vi "Move_Copy.vi"(1 "Mode":enum16{"Move", "Copy"}(ring), 2 "Send error message?":bool=TRUE, 3 "Only Local Copy?":bool, 4 "target path":path, 6 "source path":path) -> ()   [LabVIEW 2010]
uses:
  Update_Global.vi
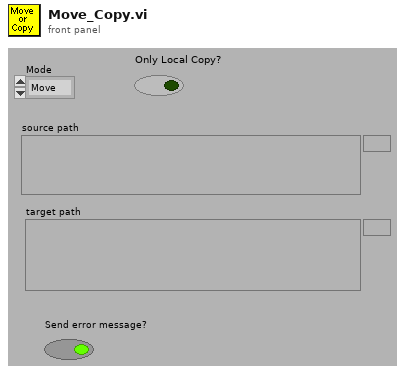
[diagram p1: front panel]
types:
  T1 = enum16{"read/write", "read-only", "write-only", "write-only (truncate)"}
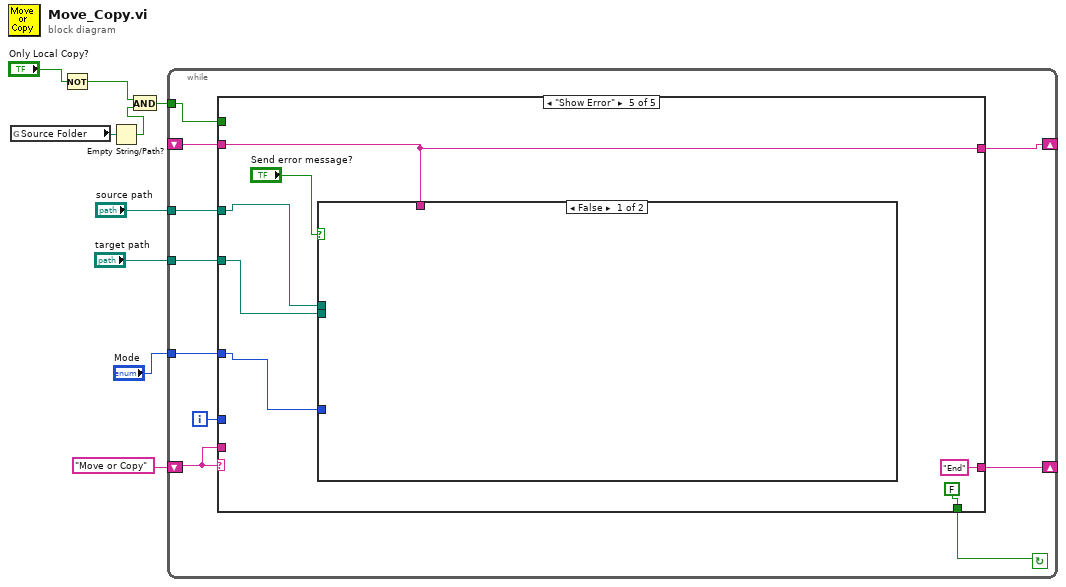
[diagram p0: block diagram]
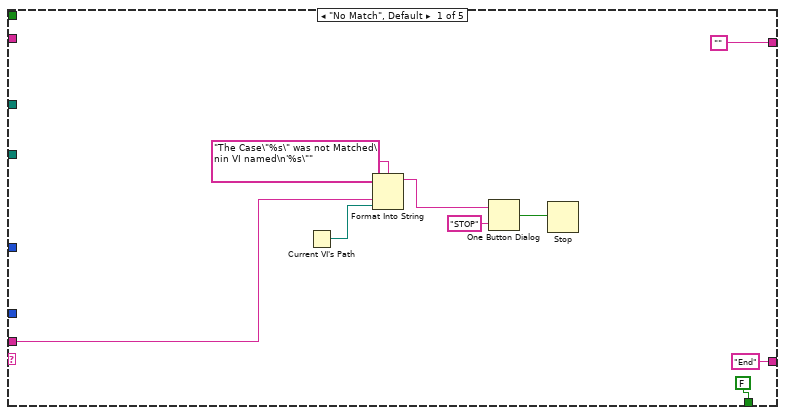
[diagram p2: hidden frame]
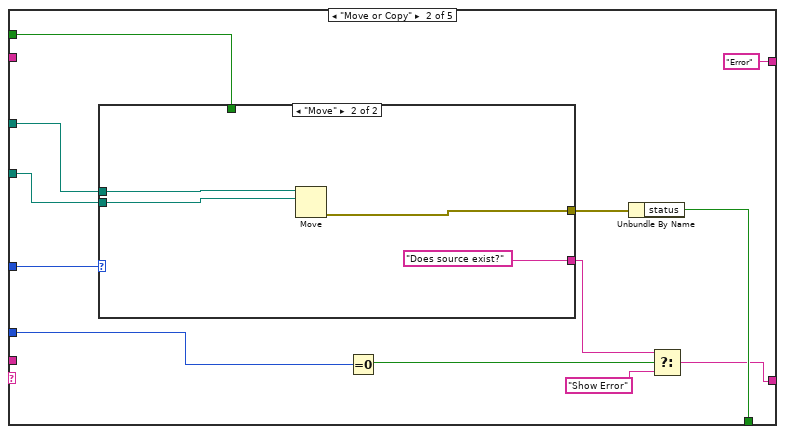
[diagram p3: hidden frame]
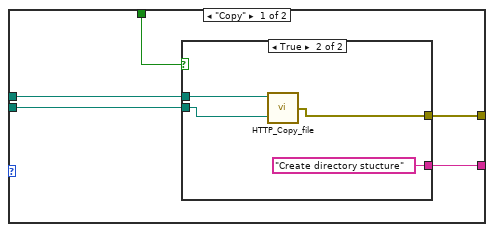
[diagram p4: hidden frame]
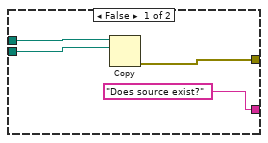
[diagram p5: hidden frame]
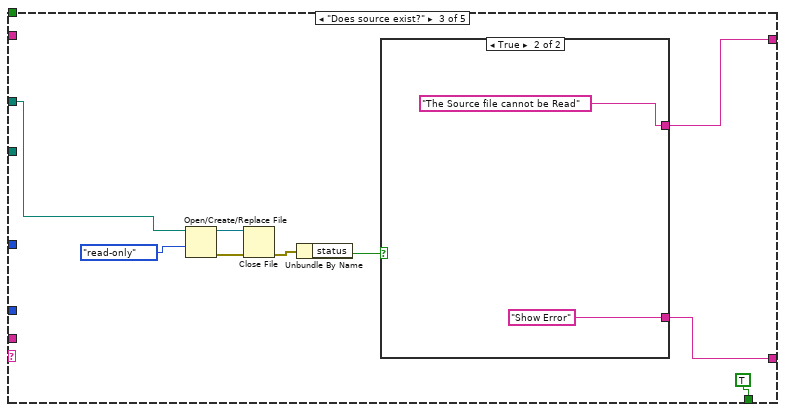
[diagram p6: hidden frame]
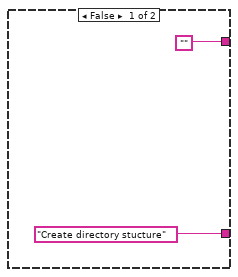
[diagram p7: hidden frame]
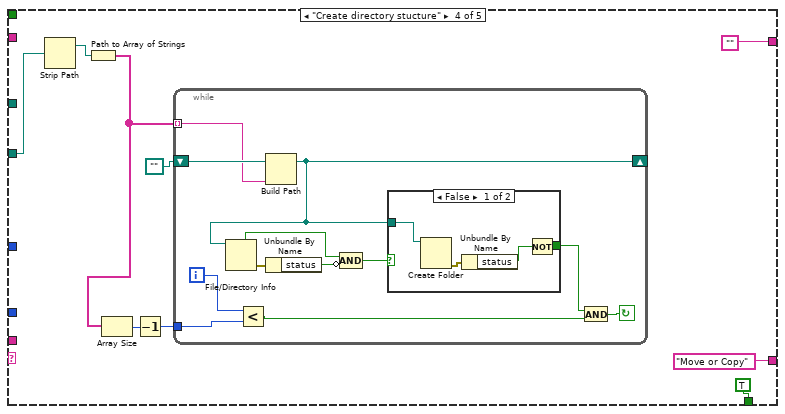
[diagram p8: hidden frame]
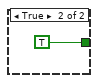
[diagram p9: hidden frame]
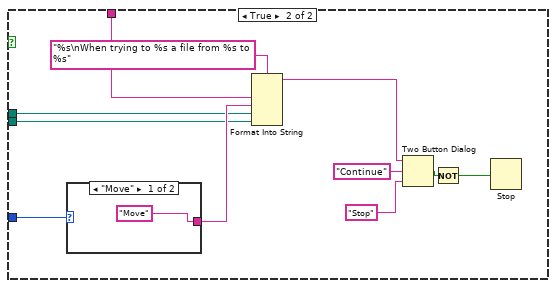
[diagram p10: hidden frame]
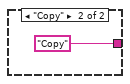
[diagram p11: hidden frame]
diagram:
  n1 = global read "Update_Global.vi" "Source Folder"() -> (w6:path)
  n2 = Not(x="Only Local Copy?") -> (.not. x?=w2:bool)
  n3 = Empty String/Path?(string/path=w6) -> (empty?=w4:bool)
  n4 = And(x=w2, y=w4) -> (x .and. y?=w3:bool)
  n5 = while {
    shift-left: "Move or Copy" -> [w10]
    shift-right: [w19] -> _
    tunnel: "source path" -> [w17]
    tunnel: "target path" -> [w16]
    tunnel: "Mode" -> [w15]
    tunnel: w3 -> [w13]
    shift-right: [w11] -> _
    shift-left: _ -> [w12]
    i -> [w14]
    stop <- w18 continue-if-true
    n6 = case shown="\"Show Error\"" w10 {
      tunnel: ["End" ("f") w30 w60 "Move or Copy" "End" ("f")] -> w19
      tunnel: [FALSE ("status") w34 TRUE ("status") TRUE FALSE ("status")] -> w18
      tunnel: w17 -> [_ w40 w59 _ w99]
      tunnel: w16 -> [_ w39 _ w74 w98]
      tunnel: w15 -> [_ w38 _ _ w103]
      tunnel: w14 -> [_ w37 _ _ _]
      tunnel: w13 -> [_ w35 _ _ _]
      tunnel: w12 -> [_ _ _ _ w100]
      tunnel: ["" "Error" ("format string") w58 "" w100] -> w11
      tunnel: w10 -> [w23 _ _ _ _]
      frame "No Match", Default {
        n7 = Current VI's Path() -> (path=w28:path)
        n8 = Format Into String(format string="The Case\"%s\" was not Matched\nin VI named\n'%s\"" ("Format String"), w23, w28) -> (resulting string=w25:string)  [unwired: 2 in, 1 out]
        n9 = One Button Dialog(message=w25, button name ("OK")="STOP") -> (true=w27:bool)
        n10 = Stop(stop? (T)=w27) -> ()
      }
      frame "Move or Copy" {
        n11 = case shown="\"Move\"" w38 {
          tunnel: w40 -> [w45 w57]
          tunnel: w39 -> [w44 w56]
          tunnel: [w43 w55] -> w36
          tunnel: w35 -> [w42 _]
          tunnel: [w41 "Does source exist?"] -> w32
          frame "Copy" {
            n12 = case shown="True" w42 {
              tunnel: w45 -> [w49 w53]
              tunnel: w44 -> [w48 w52]
              tunnel: [w47 w51] -> w43
              tunnel: ["Does source exist?" "Create directory stucture"] -> w41
              frame False {
                n13 = Copy(10:w48, 11:w49) -> (0:w47:errorcluster)  [unwired: 1 in, 4 out]
              }
              frame True {
                n14 = call "HTTP_Copy_file.vi"("target path"=w52, "Source Path"=w53) -> ("error out"=w51:errorcluster)
              }
            }
          }
          frame "Move" {
            n15 = Move(source path=w57, 10:w56) -> (error out=w55:errorcluster)  [unwired: 1 in, 4 out]
          }
        }
        n16 = Equal To 0?(x=w37) -> (x = 0?=w33:bool)
        n17 = Unbundle By Name(w36) -> ("status"=w34:bool)
        n18 = Select(t=w32, s=w33, f="Show Error") -> (s? t:f=w30:string)
      }
      frame "Does source exist?" {
        n19 = Open/Create/Replace File(file path (use dialog)=w59, access (0:read/write)=T1."read-only" ("open mode (0)")) -> (refnum out=w64:refnum<file>, error out=w66:errorcluster)  [unwired: 1 in, 4 out]
        n20 = Close File(refnum=w64, error in=w66) -> (error out=w63:errorcluster)  [unwired: 1 out]
        n21 = Unbundle By Name(w63) -> ("status"=w61:bool)
        n22 = case shown="True" w61 {
          tunnel: ["Create directory stucture" ("f") "Show Error" ("f")] -> w60
          tunnel: ["" "The Source file cannot be Read" ("format string")] -> w58
          frame False {
          }
          frame True {
          }
        }
      }
      frame "Create directory stucture" {
        n23 = Strip Path(path=w74) -> (stripped path=w73:path)  [unwired: 1 out]
        n24 = Path to Array of Strings(0:w73) -> (2:w76:string[])  [unwired: 1 out]
        n25 = Array Size(array=w76) -> (size(s)=w77:i32)
        n26 = Decrement(x=w77) -> (x-1=w78:i32)
        n27 = while {
          tunnel: w78 -> [w88]
          shift-left: path "" ("appended path") -> [w91]
          shift-right: [w85] -> _
          tunnel: w76 -> [w90] mode=indexing
          i -> [w89]
          stop <- w86 continue-if-true
          n28 = Less?(x=w89, y=w88) -> (x < y?=w87:bool)
          n29 = Build Path(base path=w91, name or relative path=w90) -> (appended path=w85:path)
          n30 = File/Directory Info(path=w85) -> (directory=w82:bool, error out=w84:errorcluster)  [unwired: 1 in, 5 out]
          n31 = Unbundle By Name(w84) -> ("status"=w83:bool)
          n32 = Compound Arithmetic op=AND(w82, invert w83) -> (w81:bool)
          n33 = case shown="False" w81 {
            tunnel: w85 -> [w95 _]
            tunnel: [w92 TRUE] -> w80
            frame False {
              n34 = Create Folder(path (use dialog)=w95) -> (error out=w94:errorcluster)  [unwired: 1 in, 3 out]
              n35 = Unbundle By Name(w94) -> ("status"=w93:bool)
              n36 = Not(x=w93) -> (.not. x?=w92:bool)
            }
            frame True {
            }
          }
          n37 = And(x=w80, y=w87) -> (x .and. y?=w86:bool)
        }
      }
      frame "Show Error" {
        n38 = case shown="False" "Send error message?" {
          tunnel: w103 -> [_ w110]
          tunnel: w100 -> [_ w109]
          tunnel: w99 -> [_ w106]
          tunnel: w98 -> [_ w105]
          frame False {
          }
          frame True {
            n39 = case shown="\"Move\"" w110 {
              tunnel: ["Move" "Copy"] -> w108
              frame "Move" {
              }
              frame "Copy" {
              }
            }
            n40 = Format Into String(format string="%s\nWhen trying to %s a file from %s to %s", w109, w108, w106, w105) -> (resulting string=w104:string)  [unwired: 2 in, 1 out]
            n41 = Two Button Dialog(message=w104, 1:"Stop" ("F button name (\"Cancel\")"), 2:"Continue" ("T button name (\"OK\")")) -> (T button?=w114:bool)
            n42 = Not(x=w114) -> (.not. x?=w113:bool)
            n43 = Stop(stop? (T)=w113) -> ()
          }
        }
      }
    }
  }
